vi "GetCurrentYYYYMMDDString.vi"(11 "displayTime":timestamp) -> (3 "data":T1)   [LabVIEW 2017, in "UI_TimeSelector.xctl"]
uses:
  UI_TimeSelector/UI_TimeSelector.xctl
  UI_TimeSelector/Typedefs/INTERNAL-DATA.ctl
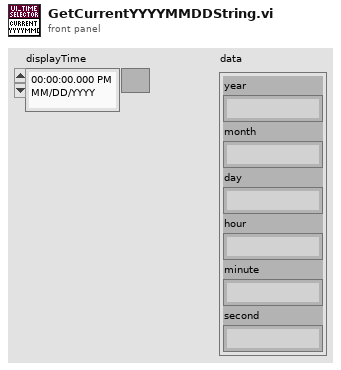
[diagram p1: front panel]
types:
  T1 = typedef "UI_TimeSelector.xctl/INTERNAL-DATA.ctl" = cluster{"year":string, "month":string, "day":string, "hour":string, "minute":string, "second":string}
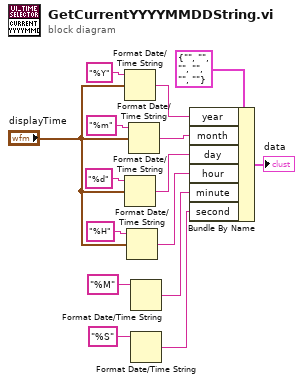
[diagram p0: block diagram]
diagram:
  n1 = Format Date/Time String(time format string (%c)="%Y", seconds (now)="displayTime") -> (date/time string=w1:string)  [unwired: 1 in]
  n2 = Format Date/Time String(time format string (%c)="%d", seconds (now)="displayTime") -> (date/time string=w3:string)  [unwired: 1 in]
  n3 = Format Date/Time String(time format string (%c)="%H", seconds (now)="displayTime") -> (date/time string=w4:string)  [unwired: 1 in]
  n4 = Format Date/Time String(time format string (%c)="%m", seconds (now)="displayTime") -> (date/time string=w2:string)  [unwired: 1 in]
  n5 = Format Date/Time String(time format string (%c)="%M") -> (date/time string=w5:string)  [unwired: 2 in]
  n6 = Format Date/Time String(time format string (%c)="%S") -> (date/time string=w6:string)  [unwired: 2 in]
  n7 = Bundle By Name(cluster=T1 {"year"="", "month"="", "day"="", "hour"="", "minute"="", "second"=""} ("data"), "year"=w1, "month"=w2, "day"=w3, "hour"=w4, "minute"=w5, "second"=w6) -> (→"data":T1)
